vi "Set Error.vi"(9 "Override":errorcluster, 10 "Merge":errorcluster, 11 "Dev Actor in":refnum<class "Dev Actor.lvclass">) -> (3 "Dev Actor out":refnum<class "Dev Actor.lvclass">)   [LabVIEW 2021, in "Dev Actor.lvlib" / "Dev Actor.lvclass"]
uses:
  Dev Actor.lvclass
  Dev Actor.lvclass/Dev Actor.ctl
  <vilib>/jettl/jettl/Actor/Actor/Actor.lvclass
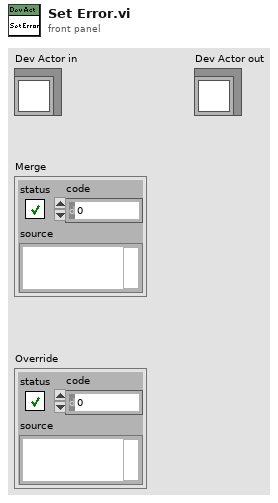
[diagram p1: front panel]
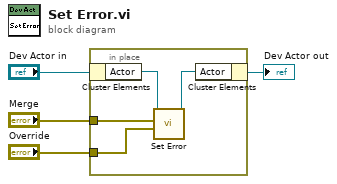
[diagram p0: block diagram]
diagram:
  n1 = in-place {
    in-place-border: "Merge" -> [w6]
    in-place-border: "Override" -> [w5]
    n2 = in-place-cluster #1("Dev Actor in") -> ("Actor"=w8:refnum<class "Actor.lvclass">)
    n3 = call-dynamic "Set Error.vi"("Override"=w5, "Merge"=w6, "Set Error in"=w8) -> ("Set Error out"=w7:refnum<class "Actor.lvclass">)  [unwired: 8 in]
    n4 = in-place-cluster #1("Actor"=w7) -> (→"Dev Actor out":refnum<class "Dev Actor.lvclass">)
  }
